vi "Test ExampleClone API.vi"() -> ()   [LabVIEW 2020]
doc: "ExampleClone API Tester.\n\n<b>Note:</b> This VI was modified by the <b>Validate DQMH Module</b> tool to add the 'Show Main VI Diagram on Init' functionality included in DQMH 6.1.\n\n<b>Note:</b> This VI was modified by the <b>Validate DQMH Module</b> tool to upgrade its Error Reported event frame to use an improved mechanism for displaying error information.\n\n____\nHAMPEL SOFTWARE ENGINEERING v2.6.0 (2023-12-19 10:54)"
uses:
  Libraries/hse-libraries/Source/hse-dqmh/Controls/Module Display Scenarios.ctl
  <vilib>/Utility/error.llb/DialogType.ctl
  <vilib>/Hampel Software Engineering/HSE Logger/LogRecord/LogRecord.lvclass/LogRecord.ctl
  ExampleClone.lvlib
  Libraries/hse-libraries/Source/hse-dqmh/hse-dqmh.lvlib
  <vilib>/Hampel Software Engineering/HSE Logger/hse-logger.lvlib
  <vilib>/Hampel Software Engineering/HSE Logger/LogRecord/LogRecord.lvclass
panel:
  in  "Show Main VI Diagram on Init (F)":bool
  in  "Scenario":T1
  in  "Request UI Display":bool
  in  "Prepare":bool
  in  "Configure":bool
  in  "ExampleMessage 2":string
  in  "ExampleMessage":bool
  in  "Run as Singleton?":bool
  in  "Show Block Diagram":bool
  in  "Refresh Modules":bool
  out "Active Modules":string[](array[string])
  in  "Stop Module":bool
  in  "Select Module":i32(ring)=-1 caption="Select Module\nTo send Request to" items=["All"=-1, "4140002"=4140002]
  in  "Run New Module":bool
  in  "Hide Module Panel":bool
  in  "Show Module Panel":bool
  out "Status":string
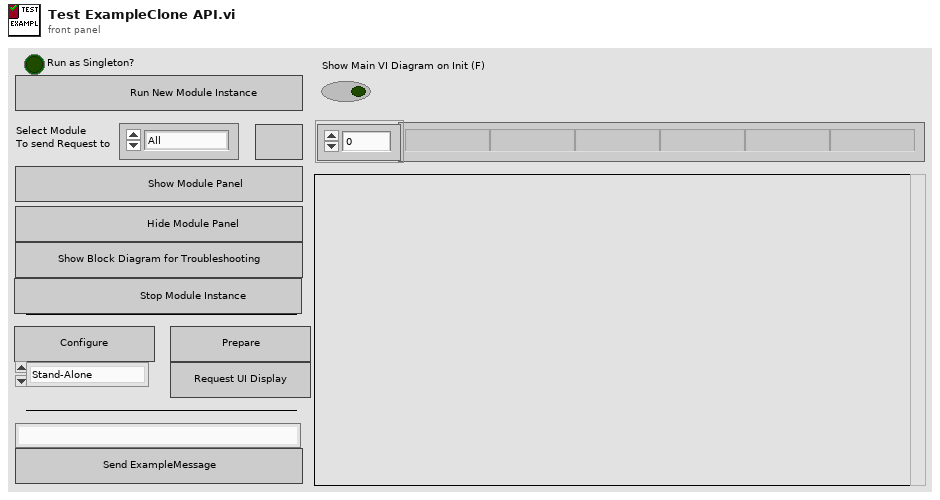
[diagram p1: front panel]
types:
  T1 = typedef "hse-dqmh.lvlib/Module Display Scenarios.ctl" = enum16{"Stand-Alone", "Managed"}
  T2 = typedef "ExampleClone.lvlib/Broadcast Events--cluster.ctl" = cluster{"Module Did Init":refnum<user-event>, "Status Updated":refnum<user-event>, "Error Reported":refnum<user-event>, "Module Did Stop":refnum<user-event>, "Update Module Execution Status":refnum<user-event>, "System Message":refnum<user-event>}
  T3 = typedef "DialogType.ctl" = u16
  T4 = typedef "hse-dqmh.lvlib/System Message Source.ctl" = enum16{"module", "application", "network"}
  T5 = typedef "hse-logger.lvlib/LogLevel.ctl" = enum16{"DEBUG", "INFO", "WARNING", "ERROR", "CRITICAL"}
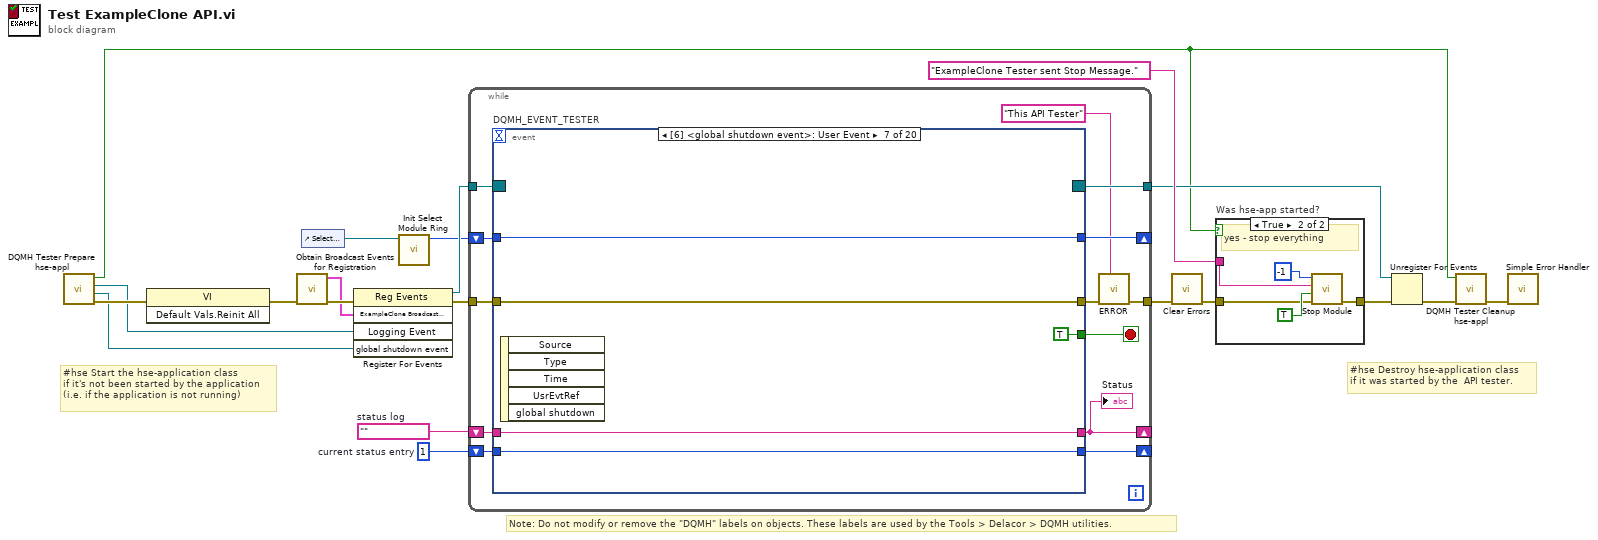
[diagram p0: block diagram]
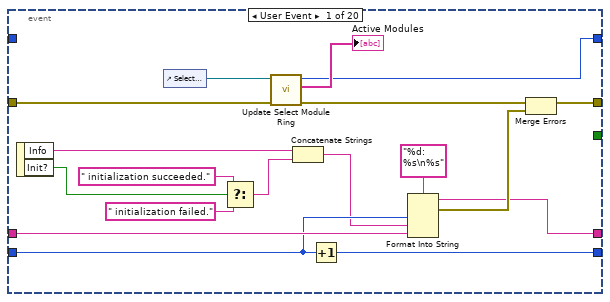
[diagram p3: hidden frame]
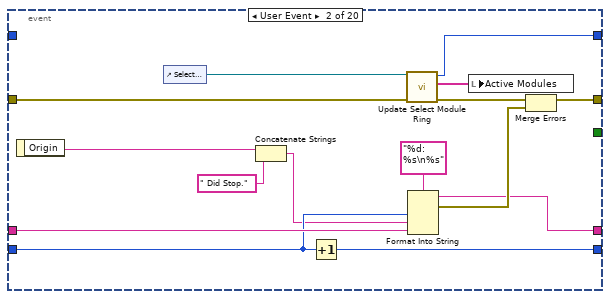
[diagram p4: hidden frame]
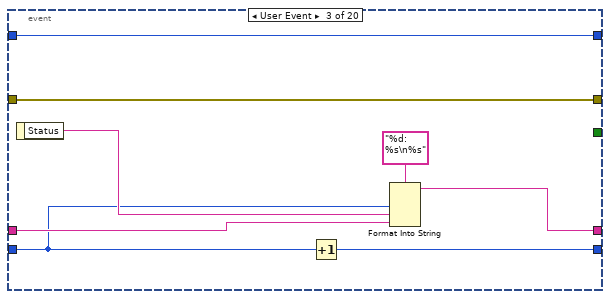
[diagram p5: hidden frame]
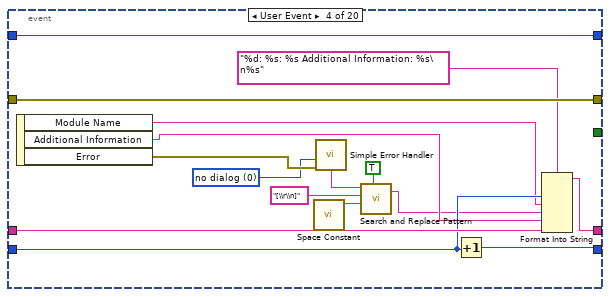
[diagram p6: hidden frame]
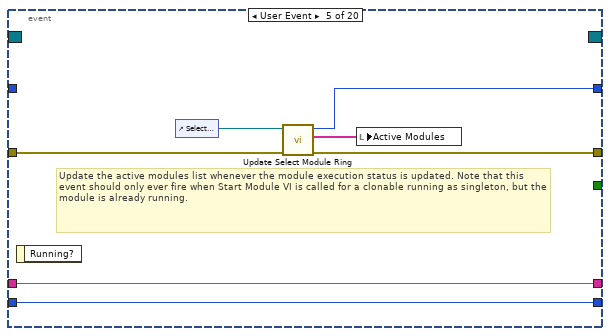
[diagram p7: hidden frame]
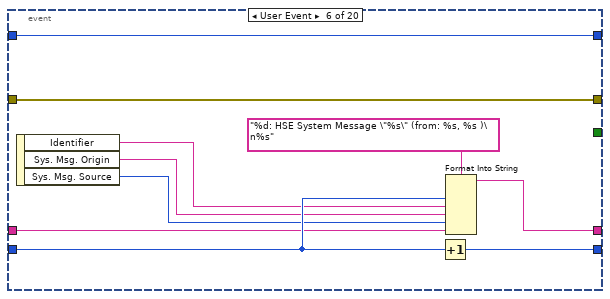
[diagram p8: hidden frame]
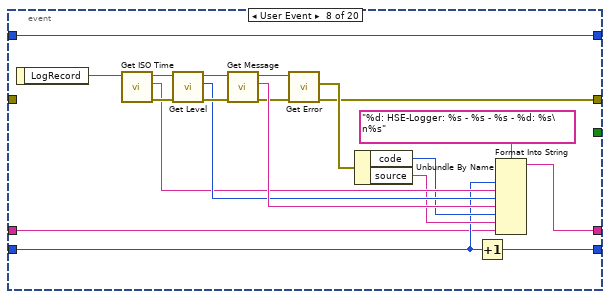
[diagram p9: hidden frame]
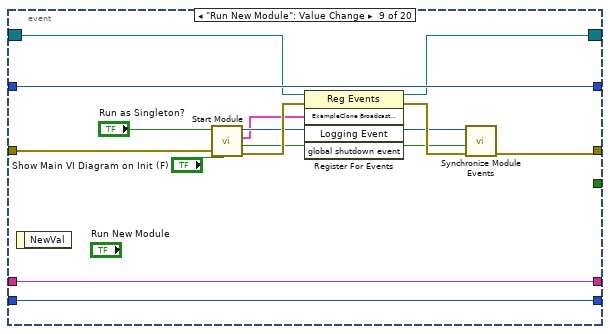
[diagram p10: hidden frame]
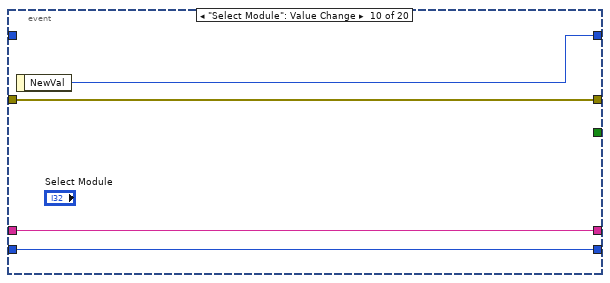
[diagram p11: hidden frame]
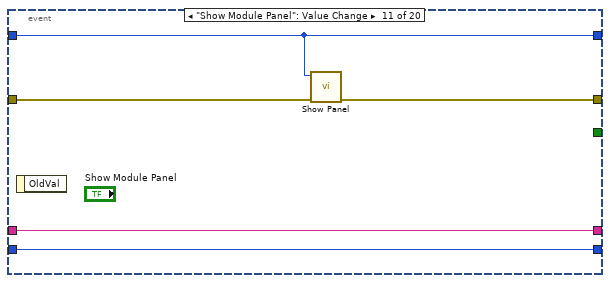
[diagram p12: hidden frame]
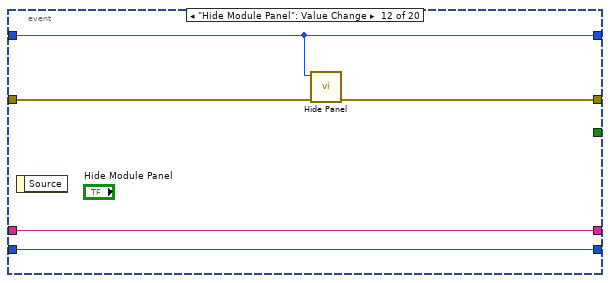
[diagram p13: hidden frame]
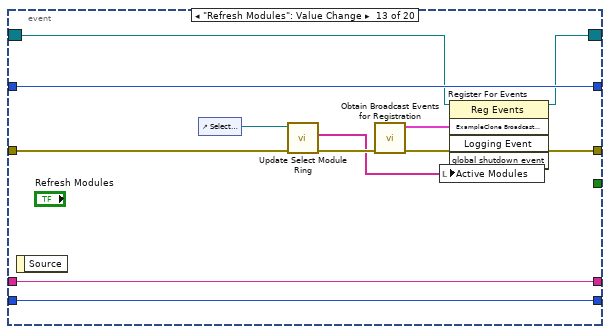
[diagram p14: hidden frame]
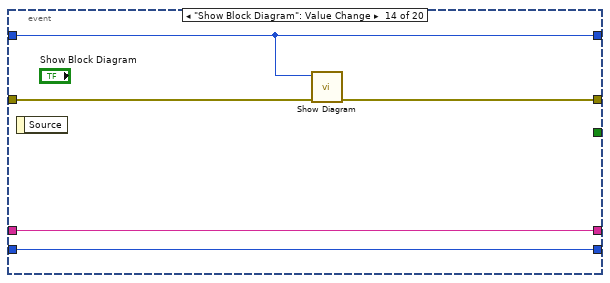
[diagram p15: hidden frame]
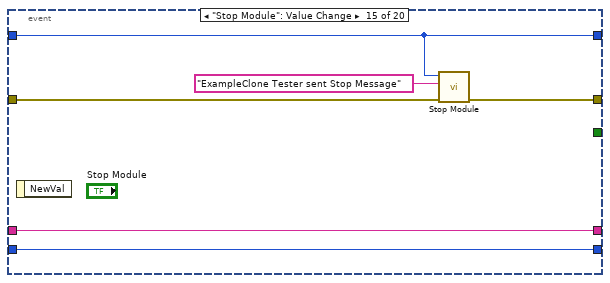
[diagram p16: hidden frame]
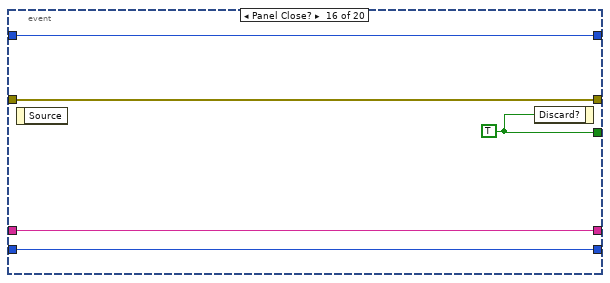
[diagram p17: hidden frame]
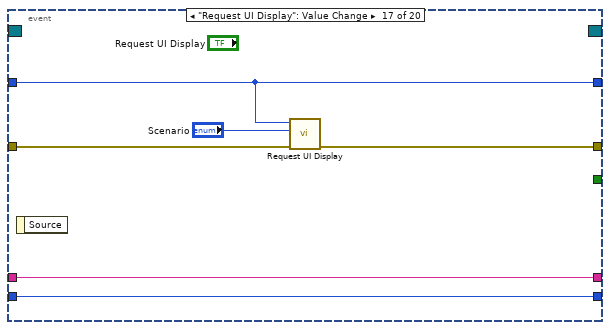
[diagram p18: hidden frame]
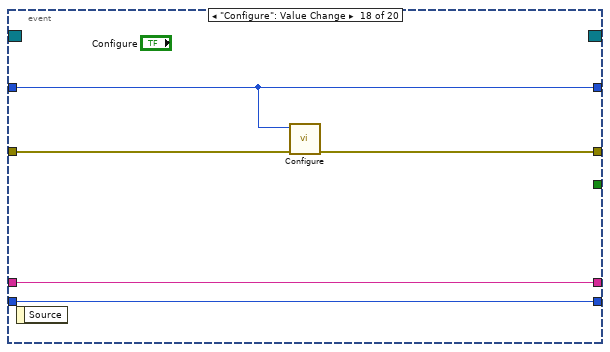
[diagram p19: hidden frame]
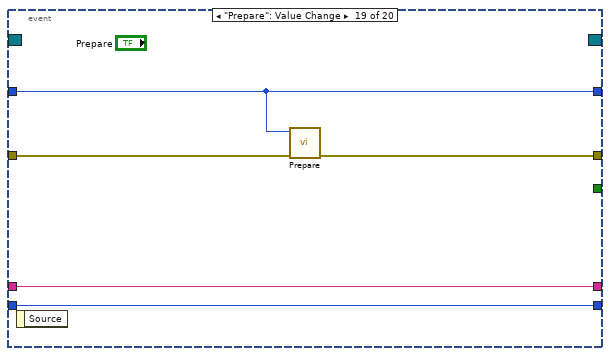
[diagram p20: hidden frame]
diagram:
  w16 = 1  # current status entry
  w17 = ""  # status log
  # "#hse Destroy hse-application class \nif it was started by the  API tester."
  # "#hse Start the hse-application class \nif it's not been started by the application\n(i.e. if the application is not running)"
  # "Note: Do not modify or remove the \"DQMH\" labels on objects. These labels are used by the Tools > Delacor > DQMH utilities."
  n1 = call "DQMH Tester Prepare hse-appl.vi"() -> ("error out"=w6:errorcluster, "global shutdown event"=w1:refnum<user-event>, "Logging Event"=w5:refnum<user-event>, "Started?"=w2:bool)  [unwired: 8 in]
  n2 = invoke class="VI" method="Default Vals.Reinit All"(error in=w6) -> (error out=w8:errorcluster)  [unwired: 2 in, 2 out]
  n3 = call "Obtain Broadcast Events for Registration.vi"("error in (no error)"=w8) -> ("error out"=w7:errorcluster, "ExampleClone Broadcast Events"=w3:T2)  [unwired: 9 in]
  n4 = control-ref of="Select Module"() -> (w14:refnum<vi>)
  n5 = register-events(error in=w7, w3, w5, w1) -> (reference out=w20:refnum<event-registration>, error out=w13:errorcluster)  [unwired: 1 in]
  n6 = call "Init Select Module Ring.vi"("Select Module Ring Ref"=w14) -> ("Value for All Modules"=w15:i32)  [unwired: 8 in, 2 out]
  n7 = while {
    tunnel: w20 -> [w33]
    tunnel: [w22] -> w9
    tunnel: w13 -> [w32]
    shift-right: [w28] -> _
    shift-left: w17 -> [w30]
    shift-right: [w29] -> _
    shift-left: w16 -> [w31]
    shift-right: [w26] -> _
    shift-left: w15 -> [w27]
    tunnel: [w25] -> w11
    stop <- w23 stop-if-true
    n8 = event "DQMH_EVENT_TESTER" shown="[6] <global shutdown event>: User Event" {
      selector: w33 -> [_ _ _ _ _ _ _ _ w140 _ _ _ w166 _ _ _ _ _ _ _]
      dyn-events: [_ _ _ _ _ _ _ _ w139 _ _ _ w165 _ _ _ _ _ _ _] -> w25
      timeout: _ -> [_ _ _ _ _ _ _ _ _ _ _ _ _ _ _ _ _ _ _ _]
      tunnel: [_ _ _ _ _ _ TRUE ("Discard?") _ _ _ _ _ _ _ _ w187 _ _ _ _] -> w23
      tunnel: [w41 w58 w74 w89 w93 w107 w112 w119 w138 w150 w154 w159 w162 w173 w178 w186 w190 w195 w200 w206] -> w24
      tunnel: w32 -> [w43 w60 w74 w89 w94 w107 w112 _ w141 w150 w155 w160 w167 w176 w179 w186 w193 w198 w203 w209]
      tunnel: w31 -> [w48 w63 w67 w86 w96 w104 w110 w117 w143 w148 w152 w157 w170 w174 w181 w184 w191 w196 w201 w207]
      tunnel: w30 -> [w49 w64 w70 w88 w97 w103 w111 w116 w144 w149 w153 w158 w171 w175 w182 w185 w192 w197 w202 w208]
      tunnel: [w46 w61 w71 w87 w97 w102 w111 w115 w144 w149 w153 w158 w171 w175 w182 w185 w192 w197 w202 w208] -> w28
      tunnel: [w47 w62 w73 w85 w96 w101 w110 w118 w143 w148 w152 w157 w170 w174 w181 w184 w191 w196 w201 w207] -> w29
      tunnel: w27 -> [_ _ w68 w90 _ w106 w109 w132 w142 _ w151 w156 w169 w172 w180 w183 w189 w194 w199 w205]
      tunnel: [w38 w55 w68 w90 w92 w106 w109 w132 w142 w147 w151 w156 w169 w172 w180 w183 w189 w194 w199 w205] -> w26
      event User Event {
        n9 = event-data() -> ("Info"=w45:string, "Init?"=w35:bool)  [unwired: 1 in]
        n10 = control-ref of="Select Module"() -> (w40:refnum<vi>)
        n11 = Select(t=" initialization succeeded.", s=w35, f=" initialization failed.") -> (s? t:f=w34:string)
        n12 = call "Update Select Module Ring.vi"("error in (no error)"=w43, "Select Module Ring Ref"=w40) -> ("error out"=w42:errorcluster, "Active Modules (Array)"=→"Active Modules":string[], "New Module Ring Value"=w38:i32)  [unwired: 7 in]
        n13 = Concatenate Strings(w45, w34) -> (w44:string)
        n14 = Increment(x=w48) -> (x+1=w47:i32)
        n15 = Format Into String(format string="%d: %s\n%s", w48, w44, w49) -> (resulting string=w46:string, error out=w51:errorcluster)  [unwired: 2 in]
        n16 = Merge Errors(w42, w51) -> (w41:errorcluster)
      }
      event User Event {
        n17 = event-data() -> ("Origin"=w53:string)  [unwired: 1 in]
        n18 = control-ref of="Select Module"() -> (w57:refnum<vi>)
        n19 = Concatenate Strings(w53, " Did Stop.") -> (w52:string)
        n20 = Increment(x=w63) -> (x+1=w62:i32)
        n21 = call "Update Select Module Ring.vi"("error in (no error)"=w60, "Select Module Ring Ref"=w57) -> ("error out"=w59:errorcluster, "Active Modules (Array)"=w56:string[], "New Module Ring Value"=w55:i32)  [unwired: 7 in]
        n22 = Format Into String(format string="%d: %s\n%s", w63, w52, w64) -> (resulting string=w61:string, error out=w66:errorcluster)  [unwired: 2 in]
        n23 = local write "Active Modules"(w56) -> ()
        n24 = Merge Errors(w59, w66) -> (w58:errorcluster)
      }
      event User Event {
        n25 = event-data() -> ("Status"=w69:string)  [unwired: 1 in]
        n26 = Increment(x=w67) -> (x+1=w73:i32)
        n27 = Format Into String(format string="%d: %s\n%s", w67, w69, w70) -> (resulting string=w71:string)  [unwired: 2 in, 1 out]
      }
      event User Event {
        w81 = T3 0 items=["no dialog", "OK message", "continue or stop message", "OK message + warnings", "continue/stop + warnings"] ("type of dialog (OK msg:1)")
        n28 = event-data() -> ("Module Name"=w82:string, "Additional Information"=w83:string, "Error"=w84:errorcluster)  [unwired: 1 in]
        n29 = call <vilib>:"Space Constant.vi"() -> ("String"=w77:string)
        n30 = call <vilib>:"Simple Error Handler.vi"("type of dialog (OK msg:1)"=w81, "error in (no error)"=w84) -> ("message"=w80:string)  [unwired: 3 in, 4 out]
        n31 = call <vilib>:"Search and Replace Pattern.vi"("string"=w80, "regular expression (\"\")"="[\\r\\n]" ("regular expression (\"\")"), "replace string (\"\")"=w77, "replace all? (F)"=TRUE ("replace all CR/LF with spaces")) -> ("result string"=w79:string)  [unwired: 1 in, 1 out]
        n32 = Increment(x=w86) -> (x+1=w85:i32)
        n33 = Format Into String(format string="%d: %s: %s Additional Information: %s\n%s", w86, w82, w79, w83, w88) -> (resulting string=w87:string)  [unwired: 2 in, 1 out]
      }
      event User Event {
        # "Update the active modules list whenever the module execution status is updated. Note that this event should only ever fire when Start Module VI is called for a clonable running as singleton, but the module is already running."
        n34 = event-data() -> ()  [unwired: 1 in, 1 out]
        n35 = control-ref of="Select Module"() -> (w95:refnum<vi>)
        n36 = call "Update Select Module Ring.vi"("error in (no error)"=w94, "Select Module Ring Ref"=w95) -> ("error out"=w93:errorcluster, "Active Modules (Array)"=w91:string[], "New Module Ring Value"=w92:i32)  [unwired: 7 in]
        n37 = local write "Active Modules"(w91) -> ()
      }
      event User Event {
        n38 = event-data() -> ("Identifier"=w98:string, "Sys. Msg. Origin"=w99:string, "Sys. Msg. Source"=w100:T4)  [unwired: 1 in]
        n39 = Increment(x=w104) -> (x+1=w101:i32)
        n40 = Format Into String(format string="%d: HSE System Message \"%s\" (from: %s, %s )\n%s", w104, w98, w99, w100, w103) -> (resulting string=w102:string)  [unwired: 2 in, 1 out]
      }
      event User Event {
        n41 = event-data() -> ()  [unwired: 1 in, 5 out]
      }
      event User Event {
        n42 = event-data() -> ("LogRecord"=w113:refnum<class "LogRecord.lvclass">)  [unwired: 1 in]
        n43 = call <vilib>:"Get ISO Time.vi"("LogRecord in"=w113) -> ("error out"=w123:errorcluster, "ISO Time"=w122:string, "LogRecord out"=w125:refnum<class "LogRecord.lvclass">)  [unwired: 8 in]
        n44 = call <vilib>:"Get Level.vi"("error in"=w123, "LogRecord in"=w125) -> ("error out"=w126:errorcluster, "Level"=w124:T5, "LogRecord out"=w127:refnum<class "LogRecord.lvclass">)  [unwired: 7 in]
        n45 = call <vilib>:"Get Message.vi"("error in"=w126, "LogRecord in"=w127) -> ("error out"=w128:errorcluster, "Message"=w131:string, "LogRecord out"=w129:refnum<class "LogRecord.lvclass">)  [unwired: 7 in]
        n46 = call <vilib>:"Get Error.vi"("error in"=w128, "LogRecord in"=w129) -> ("error out"=w119:errorcluster, "Error"=w130:errorcluster)  [unwired: 7 in, 1 out]
        n47 = Unbundle By Name(w130) -> ("code"=w120:i32, "source"=w121:string)
        n48 = Increment(x=w117) -> (x+1=w118:i32)
        n49 = Format Into String(format string="%d: HSE-Logger: %s - %s - %s - %d: %s\n%s", w117, w122, w124, w131, w120, w121, w116) -> (resulting string=w115:string)  [unwired: 2 in, 1 out]
      }
      event "Run New Module": Value Change {
        n50 = event-data() -> ()  [unwired: 1 in, 1 out]
        n51 = call "Start Module.vi"("Show Main VI Diagram on Init (F)"="Show Main VI Diagram on Init (F)", "error in (no error)"=w141, "Run as Singleton? (F)"="Run as Singleton?") -> ("error out"=w145:errorcluster, "Wait for Event Sync?"=w136:bool, "ExampleClone Broadcast Events"=w135:T2, "Module ID"=w137:i32)  [unwired: 5 in]
        n52 = register-events(reference=w140, error in=w145, w135) -> (reference out=w139:refnum<event-registration>, error out=w146:errorcluster)  [unwired: 2 in]
        n53 = call "Synchronize Module Events.vi"("error in (no error)"=w146, "Wait for Event Sync?"=w136, "Module ID"=w137) -> ("error out"=w138:errorcluster)  [unwired: 7 in, 1 out]
      }
      event "Select Module": Value Change {
        n54 = event-data() -> ("NewVal"=w147:i32)  [unwired: 1 in]
      }
      event "Show Module Panel": Value Change {
        n55 = event-data() -> ()  [unwired: 1 in, 1 out]
        n56 = call "Show Panel.vi"("error in (no error)"=w155, "Module ID"=w151) -> ("error out"=w154:errorcluster)  [unwired: 9 in]
      }
      event "Hide Module Panel": Value Change {
        n57 = event-data() -> ()  [unwired: 1 in, 1 out]
        n58 = call "Hide Panel.vi"("error in (no error)"=w160, "Module ID"=w156) -> ("error out"=w159:errorcluster)  [unwired: 9 in]
      }
      event "Refresh Modules": Value Change {
        n59 = event-data() -> ()  [unwired: 1 in, 1 out]
        n60 = control-ref of="Select Module"() -> (w168:refnum<vi>)
        n61 = call "Update Select Module Ring.vi"("error in (no error)"=w167, "Select Module Ring Ref"=w168) -> ("error out"=w163:errorcluster, "Active Modules (Array)"=w161:string[])  [unwired: 7 in, 1 out]
        n62 = call "Obtain Broadcast Events for Registration.vi"("error in (no error)"=w163) -> ("error out"=w162:errorcluster, "ExampleClone Broadcast Events"=w164:T2)  [unwired: 9 in]
        n63 = local write "Active Modules"(w161) -> ()
        n64 = register-events(reference=w166, w164) -> (reference out=w165:refnum<event-registration>)  [unwired: 3 in, 1 out]
      }
      event "Show Block Diagram": Value Change {
        n65 = event-data() -> ()  [unwired: 1 in, 1 out]
        n66 = call "Show Diagram.vi"("error in (no error)"=w176, "Module ID"=w172) -> ("error out"=w173:errorcluster)  [unwired: 9 in]
      }
      event "Stop Module": Value Change {
        n67 = event-data() -> ()  [unwired: 1 in, 1 out]
        n68 = call "Stop Module.vi"("error in (no error)"=w179, "Origin"="ExampleClone Tester sent Stop Message", "Module ID"=w180) -> ("error out"=w178:errorcluster)  [unwired: 8 in]
      }
      event Panel Close? {
        w187 = TRUE ("Discard?")
        n69 = event-data() -> ()  [unwired: 1 in, 1 out]
        n70 = event-data("Discard?"=w187) -> ()  [unwired: 1 in, 1 out]
      }
      event "Request UI Display": Value Change {
        n71 = event-data() -> ()  [unwired: 1 in, 1 out]
        n72 = call "Request UI Display.vi"("error in (no error)"=w193, "Scenario"="Scenario", "Module ID"=w189) -> ("error out"=w190:errorcluster)  [unwired: 7 in, 1 out]
      }
      event "Configure": Value Change {
        n73 = event-data() -> ()  [unwired: 1 in, 1 out]
        n74 = call "Configure.vi"("error in (no error)"=w198, "Module ID"=w194) -> ("error out"=w195:errorcluster)  [unwired: 9 in]
      }
      event "Prepare": Value Change {
        n75 = event-data() -> ()  [unwired: 1 in, 1 out]
        n76 = call "Prepare.vi"("error in (no error)"=w203, "Module ID"=w199) -> ("error out"=w200:errorcluster)  [unwired: 9 in]
      }
      event "ExampleMessage": Value Change {
        n77 = event-data() -> ()  [unwired: 1 in, 1 out]
        n78 = call "ExampleMessage.vi"("error in (no error)"=w209, "ExampleMessage"="ExampleMessage 2", "Module ID"=w205) -> ("error out"=w206:errorcluster)  [unwired: 8 in]
      }
    }
    "Status" <- w28
    n79 = call <vilib>:"ERROR.vi"("Message"="This API Tester" ("Origin"), "error in"=w24) -> ("error out"=w22:errorcluster)  [unwired: 9 in]
  }
  n80 = call <vilib>:"Clear Errors.vi"("error in (no error)"=w9) -> ("error out"=w10:errorcluster)  [unwired: 5 in, 1 out]
  n81 = case "Was hse-app started?" shown="True" w2 {
    tunnel: [w210 w215] -> w18
    tunnel: "ExampleClone Tester sent Stop Message." ("Origin") -> [_ w214]
    tunnel: w10 -> [w210 w211]
    frame False {
      # "no - leave all in place"
    }
    frame True {
      # "yes - stop everything"
      n82 = call "Stop Module.vi"("error in (no error)"=w211, "Wait for Module to stop? (F)"=TRUE ("Wait for Module to stop?"), "Origin"=w214, "Module ID"=-1 ("Stop all")) -> ("error out"=w215:errorcluster)  [unwired: 7 in]
    }
  }
  n83 = Unregister For Events(event registration refnum=w11, error in=w18) -> (error out=w19:errorcluster)
  n84 = call "DQMH Tester Cleanup hse-appl.vi"("error in"=w19, "Stop?"=w2) -> ("error out"=w4:errorcluster)  [unwired: 9 in]
  n85 = call <vilib>:"Simple Error Handler.vi"("error in (no error)"=w4) -> ()  [unwired: 4 in, 5 out]
